vi "Model 135 via GPIB.vi"(3 "error in":T1, 4 "GPIB Setup":cluster{"GPIB address":i16, "GPIB bus":i16}={"GPIB address"=1, "GPIB bus"=0}, 5 "Configuration In":T2={"Sensor Length (cm)"=100.0, "Hi Setpoint (cm)"=80.0, "Lo Setpoint (cm)"=20.0, "Sampling Interval (min)"=1.0} {"Sampling Interval (min)" min=0 max=600 format="%.1f"; "Lo Setpoint (cm)" min=0 max=203.2 format="%.1f"; "Hi Setpoint (cm)" min=0 max=203.2 format="%.1f"; "Sensor Length (cm)" min=1 max=203.2 format="%.1f"}, 6 "Perform\nInitialization?:F":bool) -> (0 "error out":T1={"error"=TRUE, "code"=14, "source"="Send in \u0000GPIB Command.vi->Set Coil Constant.vi->Field, Temp, and Level Example.vi"}, 1 "Configuration Out":T2={"Sensor Length (cm)"=100.0, "Hi Setpoint (cm)"=80.0, "Lo Setpoint (cm)"=20.0, "Sampling Interval (min)"=1.0} {"Sampling Interval (min)" min=0 max=600 format="%.1f"; "Lo Setpoint (cm)" min=0 max=203.2 format="%.1f"; "Hi Setpoint (cm)" min=0 max=203.2 format="%.1f"; "Sensor Length (cm)" min=1 max=203.2 format="%.1f"}, 2 "Display":sgl format="%.1f")   [LabVIEW 2013]
doc: "This is the virtual control panel for the Model 135 instrument. You should scroll to the area above the instrument to set the initialization method, communication parameters, and the initial instrument state (if not initializing from the instrument) before starting the VI. See the provided printed documentation for more information on operating the virtual instrument."
panel:
  in  "Case Constant\n(See Context Help)":bool=TRUE
  in  "Continuous/Sample Switch":bool
  out "Power LED":bool
  out "Lo LED":bool
  out "Hi LED":bool
  in  "Initialize State from Instrument?":bool
  in  "Power":bool=TRUE
  in  "Counts (hidden)":i16
  out "Query LED":bool
  in  "Rotary switch":i16(knob)=2 min=0 max=4 step=1 scale=0.0..4.0
  in  "Units":u16(ring)=2
  in  "Raise/lower":u16(ring)=1
  in  "Hidden Controls":T3 {"Prev Sampling Interval" format="%.1f"; "Prev Lo Setpoint" format="%.1f"; "Prev Hi Setpoint" format="%.1f"; "Prev Sensor Length" format="%.1f"; "Helium Level (cm)" format="%.1f"}
  # "Yes"
  # "No"
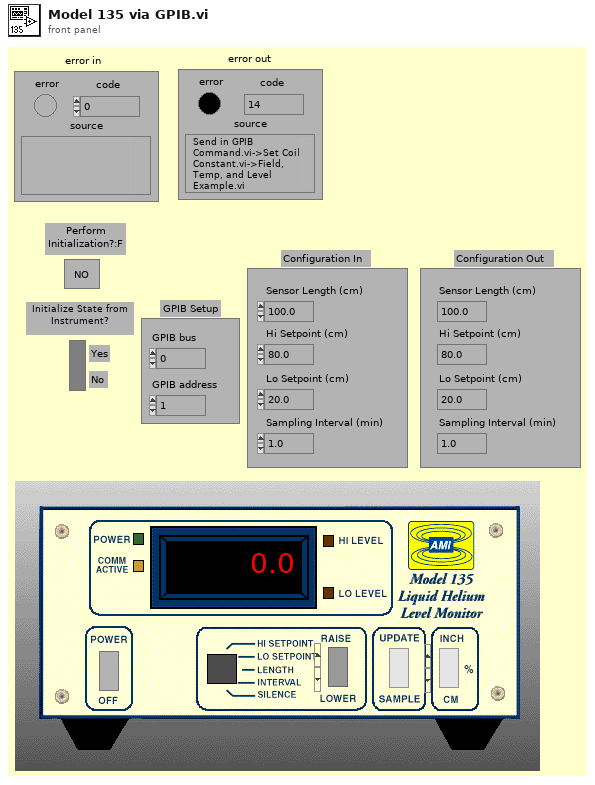
[diagram p1: front panel]
types:
  T1 = cluster{"error":bool, "code":i32, "source":string}
  T2 = cluster{"Sensor Length (cm)":sgl, "Hi Setpoint (cm)":sgl, "Lo Setpoint (cm)":sgl, "Sampling Interval (min)":sgl}
  T3 = cluster{"Helium Level (cm)":sgl, "Prev Sensor Length":sgl, "Prev Hi Setpoint":sgl, "Prev Lo Setpoint":sgl, "Prev Sampling Interval":sgl}
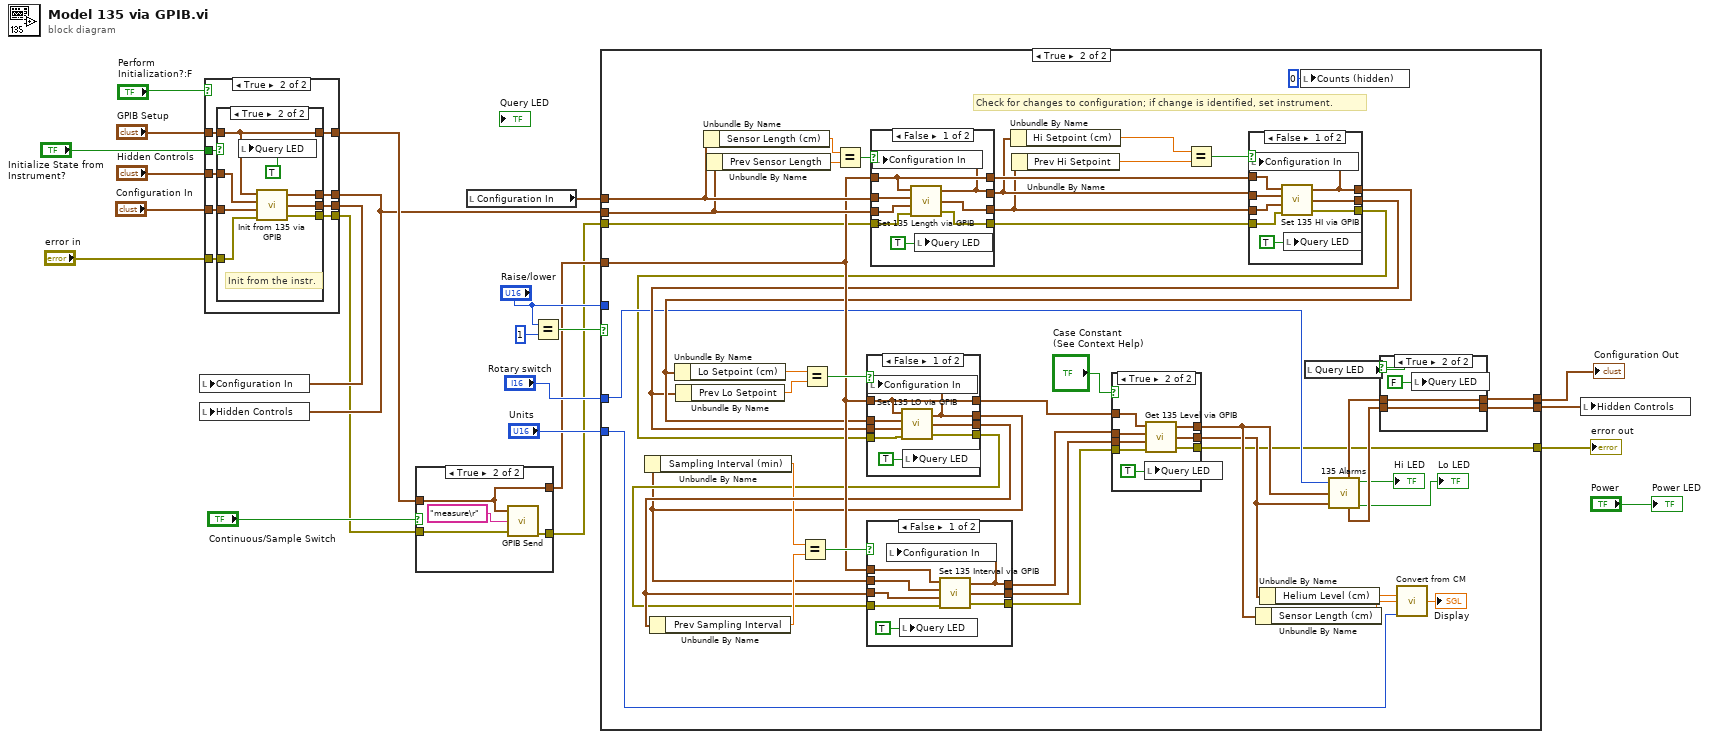
[diagram p0: block diagram]
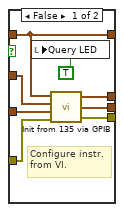
[diagram p3: hidden frame]
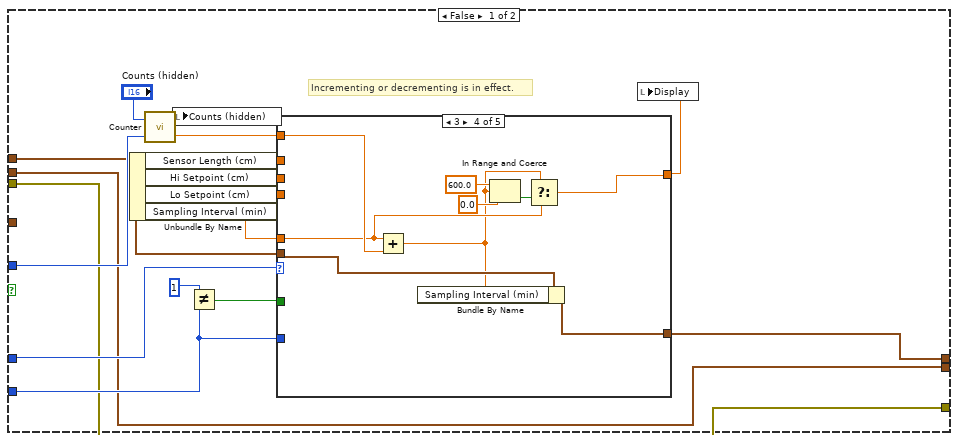
[diagram p5: hidden frame]
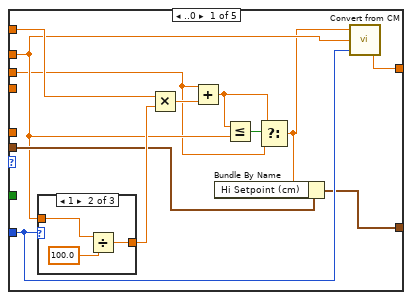
[diagram p6: hidden frame]
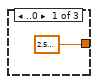
[diagram p7: hidden frame]
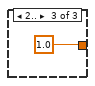
[diagram p8: hidden frame]
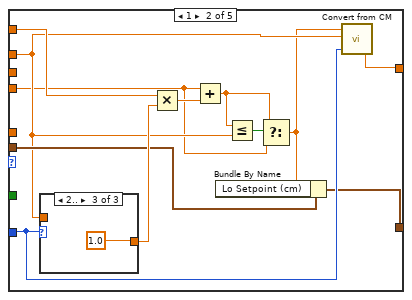
[diagram p9: hidden frame]
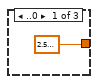
[diagram p10: hidden frame]
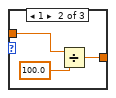
[diagram p11: hidden frame]
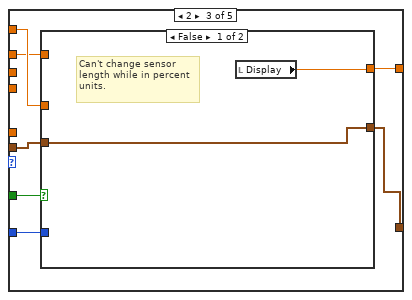
[diagram p12: hidden frame]
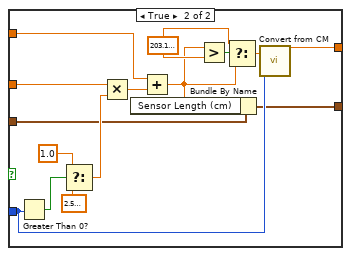
[diagram p13: hidden frame]
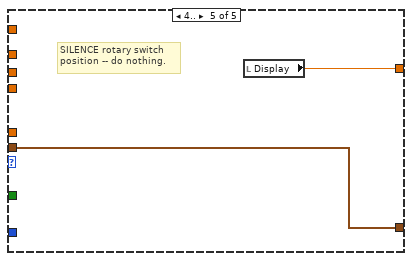
[diagram p14: hidden frame]
diagram:
  n1 = case shown="True" "Perform\nInitialization?:F" {
    tunnel: "Initialize State from Instrument?" -> [_ w36]
    tunnel: "Configuration In" -> [w25 w35]
    tunnel: "Hidden Controls" -> [w26 w34]
    tunnel: "GPIB Setup" -> [w27 w33]
    tunnel: [w27 w32] -> w19
    tunnel: [w26 w31] -> w18
    tunnel: "error in" -> [w24 w30]
    tunnel: [w25 w29] -> w4
    tunnel: [w24 w28] -> w3
    frame False {
    }
    frame True {
      n2 = case shown="True" w36 {
        tunnel: w35 -> [w42 w52]
        tunnel: w34 -> [w41 w51]
        tunnel: w33 -> [w43 w50]
        tunnel: [w43 w50] -> w32
        tunnel: [w39 w46] -> w31
        tunnel: w30 -> [w40 w48]
        tunnel: [w38 w47] -> w29
        tunnel: [w37 w45] -> w28
        frame False {
          # "Configure instr.\nfrom VI."
          n3 = local write "Query LED"(TRUE) -> ()
          n4 = call <userlib>:"Init from 135 via GPIB.vi"("error in"=w40, "Configuration (in)"=w42, "Hidden Controls (in)"=w41, "GPIB Setup"=w43) -> ("error out"=w37:T1, "Configuration (out)"=w38:T2, "Hidden Controls (out)"=w39:T3)
        }
        frame True {
          # "Init from the instr."
          n5 = local write "Query LED"(TRUE) -> ()
          n6 = call <userlib>:"Init from 135 via GPIB.vi"("error in"=w48, "Configuration (in)"=w52, "Hidden Controls (in)"=w51, "GPIB Setup"=w50) -> ("error out"=w45:T1, "Configuration (out)"=w47:T2, "Hidden Controls (out)"=w46:T3)
        }
      }
    }
  }
  n7 = local write "Configuration In"(w4) -> ()
  n8 = local write "Hidden Controls"(w18) -> ()
  n9 = case shown="True" "Continuous/Sample Switch" {
    tunnel: w19 -> [w54 w57]
    tunnel: [w54 w57] -> w11
    tunnel: w3 -> [w53 w56]
    tunnel: [w53 w55] -> w2
    frame False {
    }
    frame True {
      n10 = call <userlib>:"GPIB Send.vi"("GPIB Setup"=w57, "Input command"="measure\r", "error in"=w56) -> ("error out"=w55:T1)  [unwired: 3 out]
    }
  }
  n11 = local read "Configuration In"() -> (w9:T2)
  n12 = Equal?(x="Raise/lower", y=u16 1) -> (x = y?=w15:bool)
  n13 = case shown="True" w15 {
    tunnel: w9 -> [w66 w189]
    tunnel: w18 -> [w62 w188]
    tunnel: w11 -> [_ w163]
    tunnel: "Units" -> [w70 w157]
    tunnel: "Rotary switch" -> [w65 w158]
    tunnel: "Raise/lower" -> [w71 _]
    tunnel: [w62 w156] -> w7
    tunnel: [w59 w155] -> w17
    tunnel: w2 -> [w60 w154]
    tunnel: [w60 w146] -> w1
    frame False {
      # "Incrementing or decrementing is in effect."
      n14 = Unbundle By Name(w66) -> ("Sensor Length (cm)"=w69:sgl, "Hi Setpoint (cm)"=w64:sgl, "Lo Setpoint (cm)"=w63:sgl, "Sampling Interval (min)"=w61:sgl)
      n15 = call <userlib>:"Counter.vi"("Raise/lower"=w71, "Counts (in)"="Counts (hidden)") -> ("Multiplier"=w68:sgl, "Counts (out)"=w67:i16)
      n16 = local write "Counts (hidden)"(w67) -> ()
      n17 = Not Equal?(x=u16 1, y=w70) -> (x != y?=w74:bool)
      n18 = case shown="3" w65 {
        tunnel: [w86 w100 w115 w135 w144] -> w73
        tunnel: w68 -> [w87 w99 w116 w142 _]
        tunnel: w74 -> [_ _ w114 _ _]
        tunnel: w70 -> [w83 w98 w113 _ _]
        tunnel: w69 -> [w78 w95 w112 _ _]
        tunnel: w66 -> [w81 w97 w111 w141 w143]
        tunnel: w64 -> [w77 _ _ _ _]
        tunnel: w63 -> [_ w94 _ _ _]
        tunnel: [w79 w96 w110 w140 w143] -> w59
        tunnel: w61 -> [_ _ _ w136 _]
        frame ..0 {
          n19 = case shown="1" w83 {
            tunnel: [sgl 2.54 w90 sgl 1.0] -> w84
            tunnel: w78 -> [_ w89 _]
            frame ..0 {
            }
            frame 1 {
              n20 = Divide(x=w89, y=sgl 100.0) -> (x/y=w90:sgl)
            }
            frame 2.. {
            }
          }
          n21 = Multiply(x=w87, y=w84) -> (x*y=w85:sgl)
          n22 = Add(x=w77, y=w85) -> (x+y=w80:sgl)
          n23 = Less Or Equal?(x=w80, y=w78) -> (x <= y?=w82:bool)
          n24 = Select(t=w80, s=w82, f=w77) -> (s? t:f=w76:sgl)
          n25 = Bundle By Name(cluster=w81, "Hi Setpoint (cm)"=w76) -> (w79:T2)
          n26 = call <userlib>:"Convert from CM.vi"("Units"=w83, "Sensor Length"=w78, "Input"=w76) -> ("Output"=w86:sgl)
        }
        frame 1 {
          n27 = case shown="2.." w98 {
            tunnel: [sgl 2.54 w107 sgl 1.0] -> w103
            tunnel: w95 -> [_ w106 _]
            frame ..0 {
            }
            frame 1 {
              n28 = Divide(x=w106, y=sgl 100.0) -> (x/y=w107:sgl)
            }
            frame 2.. {
            }
          }
          n29 = Multiply(x=w99, y=w103) -> (x*y=w104:sgl)
          n30 = Add(x=w94, y=w104) -> (x+y=w101:sgl)
          n31 = Less Or Equal?(x=w101, y=w95) -> (x <= y?=w102:bool)
          n32 = Select(t=w101, s=w102, f=w94) -> (s? t:f=w93:sgl)
          n33 = Bundle By Name(cluster=w97, "Lo Setpoint (cm)"=w93) -> (w96:T2)
          n34 = call <userlib>:"Convert from CM.vi"("Units"=w98, "Sensor Length"=w95, "Input"=w93) -> ("Output"=w100:sgl)
        }
        frame 2 {
          n35 = case shown="False" w114 {
            tunnel: [w118 w132] -> w115
            tunnel: w116 -> [_ w131]
            tunnel: w113 -> [_ w125]
            tunnel: w112 -> [_ w123]
            tunnel: w111 -> [w117 w126]
            tunnel: [w117 w124] -> w110
            frame False {
              # "Can't change sensor\nlength while in percent\nunits."
              n36 = local read "Display"() -> (w118:sgl)
            }
            frame True {
              w122 = sgl 203.2
              n37 = Greater Than 0?(x=w125) -> (x > 0?=w127:bool)
              n38 = Select(t=sgl 1.0, s=w127, f=sgl 2.54) -> (s? t:f=w130:sgl)
              n39 = Multiply(x=w131, y=w130) -> (x*y=w133:sgl)
              n40 = Add(x=w123, y=w133) -> (x+y=w121:sgl)
              n41 = Bundle By Name(cluster=w126, "Sensor Length (cm)"=w121) -> (w124:T2)
              n42 = Greater?(x=w121, y=w122) -> (0:w120:bool)
              n43 = Select(t=w122, s=w120, f=w121) -> (s? t:f=w119:sgl)
              n44 = call <userlib>:"Convert from CM.vi"("Units"=w125, "Input"=w119) -> ("Output"=w132:sgl)  [unwired: 1 in]
            }
          }
        }
        frame 3 {
          n45 = Add(x=w136, y=w142) -> (x+y=w134:sgl)
          n46 = Bundle By Name(cluster=w141, "Sampling Interval (min)"=w134) -> (w140:T2)
          n47 = In Range and Coerce(upper limit=sgl 600.0, x=w134, lower limit=sgl 0.0) -> (In Range?=w139:bool)  [unwired: 1 out]
          n48 = Select(t=w134, s=w139, f=w136) -> (s? t:f=w135:sgl)
        }
        frame 4.. {
          # "SILENCE rotary switch\nposition -- do nothing."
          n49 = local read "Display"() -> (w144:sgl)
        }
      }
      n50 = local write "Display"(w73) -> ()
    }
    frame True {
      # "Check for changes to configuration; if change is identified, set instrument."
      n51 = Unbundle By Name(w189) -> ("Sensor Length (cm)"=w190:sgl)
      n52 = Unbundle By Name(w188) -> ("Prev Sensor Length"=w191:sgl)
      n53 = Equal?(x=w190, y=w191) -> (x = y?=w187:bool)
      n54 = case shown="False" w187 {
        tunnel: w189 -> [w245 w252]
        tunnel: w163 -> [w249 w253]
        tunnel: w188 -> [w244 w251]
        tunnel: [w249 w253] -> w186
        tunnel: [w246 w252] -> w185
        tunnel: [w248 w251] -> w184
        tunnel: w154 -> [w243 w250]
        tunnel: [w242 w250] -> w153
        frame False {
          n55 = call <userlib>:"Set 135 Length via GPIB.vi"("error in"=w243, "Hidden Controls (in)"=w244, "Configuration (in)"=w245, "GPIB Setup"=w249) -> ("error out"=w242:T1, "Hidden Controls (out)"=w248:T3, "Configuration (out)"=w246:T2)
          n56 = local write "Configuration In"(w246) -> ()
          n57 = local write "Query LED"(TRUE) -> ()
        }
        frame True {
        }
      }
      n58 = Unbundle By Name(w185) -> ("Hi Setpoint (cm)"=w183:sgl)
      n59 = Unbundle By Name(w184) -> ("Prev Hi Setpoint"=w182:sgl)
      n60 = Equal?(x=w183, y=w182) -> (x = y?=w181:bool)
      n61 = case shown="False" w181 {
        tunnel: w185 -> [w238 w240]
        tunnel: w186 -> [w237 _]
        tunnel: w184 -> [w236 w241]
        tunnel: [w233 w240] -> w160
        tunnel: [w235 w241] -> w159
        tunnel: w153 -> [w232 w239]
        tunnel: [w231 w239] -> w152
        frame False {
          n62 = call <userlib>:"Set 135 HI via GPIB.vi"("error in"=w232, "Hidden Controls (in)"=w236, "Configuration (in)"=w238, "GPIB Setup"=w237) -> ("error out"=w231:T1, "Hidden Controls (out)"=w235:T3, "Configuration (out)"=w233:T2)
          n63 = local write "Configuration In"(w233) -> ()
          n64 = local write "Query LED"(TRUE) -> ()
        }
        frame True {
        }
      }
      n65 = Unbundle By Name(w160) -> ("Lo Setpoint (cm)"=w175:sgl)
      n66 = Unbundle By Name(w159) -> ("Prev Lo Setpoint"=w174:sgl)
      n67 = Equal?(x=w175, y=w174) -> (x = y?=w173:bool)
      n68 = case shown="False" w173 {
        tunnel: w160 -> [w206 w213]
        tunnel: w163 -> [w210 w214]
        tunnel: w159 -> [w205 w212]
        tunnel: [w210 w214] -> w164
        tunnel: [w208 w213] -> w147
        tunnel: [w207 w212] -> w162
        tunnel: w152 -> [w204 w211]
        tunnel: [w203 w211] -> w149
        frame False {
          n69 = call <userlib>:"Set 135 LO via GPIB.vi"("error in"=w204, "Hidden Controls (in)"=w205, "Configuration (in)"=w206, "GPIB Setup"=w210) -> ("error out"=w203:T1, "Hidden Controls (out)"=w207:T3, "Configuration (out)"=w208:T2)
          n70 = local write "Configuration In"(w208) -> ()
          n71 = local write "Query LED"(TRUE) -> ()
        }
        frame True {
        }
      }
      n72 = Unbundle By Name(w147) -> ("Sampling Interval (min)"=w151:sgl)
      n73 = Unbundle By Name(w162) -> ("Prev Sampling Interval"=w166:sgl)
      n74 = Equal?(x=w151, y=w166) -> (x = y?=w165:bool)
      n75 = case shown="False" w165 {
        tunnel: w163 -> [w198 _]
        tunnel: w162 -> [w193 w201]
        tunnel: [w197 w200] -> w161
        tunnel: [w196 w201] -> w150
        tunnel: w149 -> [w195 w202]
        tunnel: [w194 w202] -> w148
        tunnel: w147 -> [w192 w200]
        frame False {
          n76 = local write "Query LED"(TRUE) -> ()
          n77 = call <userlib>:"Set 135 Interval via GPIB.vi"("error in"=w195, "Hidden Controls (in)"=w193, "Configuration (in)"=w192, "GPIB Setup"=w198) -> ("error out"=w194:T1, "Hidden Controls (out)"=w196:T3, "Configuration (out)"=w197:T2)
          n78 = local write "Configuration In"(w197) -> ()
        }
        frame True {
        }
      }
      n79 = case shown="True" "Case Constant\n(See Context Help)" {
        tunnel: [w217 w223] -> w172
        tunnel: [w216 w222] -> w171
        tunnel: w164 -> [_ w225]
        tunnel: w150 -> [w216 w220]
        tunnel: w161 -> [w217 w221]
        tunnel: w148 -> [w215 w219]
        tunnel: [w215 w218] -> w146
        frame False {
        }
        frame True {
          n80 = local write "Query LED"(TRUE) -> ()
          n81 = call <userlib>:"Get 135 Level via GPIB.vi"("error in"=w219, "Hidden Controls (in)"=w220, "Configuration (in)"=w221, "GPIB Setup"=w225) -> ("error out"=w218:T1, "Hidden Controls (out)"=w222:T3, "Configuration (out)"=w223:T2)
        }
      }
      n82 = Unbundle By Name(w172) -> ("Sensor Length (cm)"=w179:sgl)
      n83 = Unbundle By Name(w171) -> ("Helium Level (cm)"=w180:sgl)
      n84 = local write "Counts (hidden)"(i16 0) -> ()
      n85 = local read "Query LED"() -> (w177:bool)
      n86 = call <userlib>:"135 Alarms.vi"("Hidden Controls (in)"=w171, "Configuration (in)"=w172, "Rotary switch"=w158) -> ("Lo LED"=→"Lo LED":bool, "Hidden Controls (out)"=w169:T3, "Configuration (out)"=w170:T2, "Hi LED"=→"Hi LED":bool)  [unwired: 2 in]
      n87 = case shown="True" w177 {
        tunnel: w170 -> [w227 w229]
        tunnel: w169 -> [w226 w228]
        tunnel: [w227 w229] -> w155
        tunnel: [w226 w228] -> w156
        frame False {
        }
        frame True {
          n88 = local write "Query LED"(FALSE) -> ()
        }
      }
      n89 = call <userlib>:"Convert from CM.vi"("Units"=w157, "Sensor Length"=w179, "Input"=w180) -> ("Output"=→"Display":sgl)
    }
  }
  "Configuration Out" <- w17
  "error out" <- w1
  n90 = local write "Hidden Controls"(w7) -> ()
  "Power LED" <- "Power"
